vi "Make Default Model.vi"(8 "error in (no error)":errorcluster) -> (0 "error out":errorcluster, 3 "Result Model out":refnum<class "Result Model by Reference.lvclass">)   [LabVIEW 2020, in "Result Model Test Enumeration.lvclass"]
uses:
  Result Model Test Enumeration.lvclass
  source/User Interface/Result Model by Reference/Result Model by Reference.lvclass
  Result Model Test Enumeration.lvclass/Result Model Test Enumeration.ctl
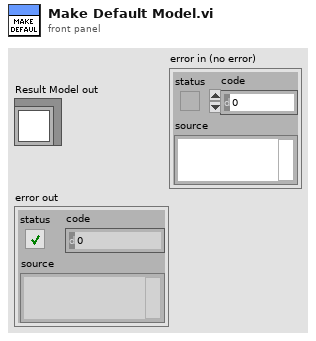
[diagram p1: front panel]
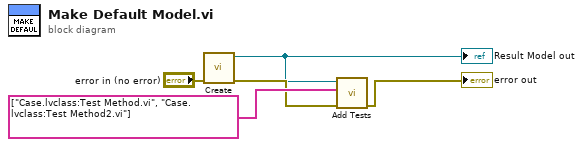
[diagram p0: block diagram]
diagram:
  n1 = call "Create.vi"("error in (no error)"="error in (no error)") -> ("error out"=w4:errorcluster, "Result Model out"=w2:refnum<class "Result Model by Reference.lvclass">)  [unwired: 9 in]
  "Result Model out" <- w2
  n2 = call "Add Tests.vi"("error in (no error)"=w4, "Tests"=string[] ["Case.lvclass:Test Method.vi", "Case.lvclass:Test Method2.vi"], "Result Model In"=w2) -> ("error out"=→"error out":errorcluster)  [unwired: 8 in]
